vi "Vehicle Position Simulation View.vi"(8 "error in (no error)":errorcluster, 11 "View Model":T1) -> (0 "error out":errorcluster)   [LabVIEW 2017]
doc: "A software interface which mimics the hardware interfaces that communicate the vehicle position.\nUsed to simulate the travel of the car through the enclosure by activating Station sensors.\n[Covers: UI4]"
uses:
  View Model/Controls/View Model.ctl
  View Model/Controls/Shared Model.ctl
  Error Handler/Controls/Error Model.ctl
  Error Handler/Controls/Error Message.ctl
  Error Handler/Controls/Error Level.ctl
  Configuration/Controls/Database Model.ctl
  Configuration/Controls/Database Message.ctl
  Configuration/Controls/Database Command.ctl
  Configuration/Controls/Database Overhead.ctl
  Configuration/Controls/Database Status.ctl
  Configuration/Controls/Database Record.ctl
  Configuration/Controls/Database - Rule Record.ctl
  Controller/Controls/CNTRLR - Wash Step.ctl
  Controller/Controls/CNTRLR - Position.ctl
  Controller/Controls/CNTRLR - Model.ctl
  Controller/Controls/CNTRLR - Message.ctl
  Controller/Controls/CNTRLR - Command.ctl
  Controller/Controls/CNTRLR - Overhead.ctl
  Controller/Controls/CNTRLR - State.ctl
panel:
  in  "Position":u32(slide) caption="Vehicle Position Simulation" max=4 scale=0.0..4.0
  # "[Covers: UI4A]"
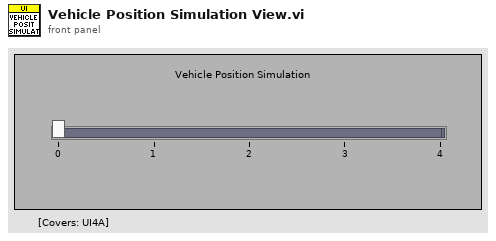
[diagram p1: front panel]
types:
  T1 = typedef "View Model.ctl" = cluster{"Shared Model":T2, "Error Model":T3, "DB Model":T4, "CNTRLR Model":T5}
  T2 = typedef "Shared Model.ctl" = cluster{"Stop":refnum<user-event>, "Stop DVR":refnum<data-value>}
  T3 = typedef "Error Model.ctl" = cluster{"Error Message":refnum<user-event>}
  T4 = typedef "Database Model.ctl" = cluster{"DB Message":refnum<user-event>, "DB Overhead DVR":refnum<data-value>}
  T5 = typedef "CNTRLR - Model.ctl" = cluster{"Message":refnum<user-event>, "Overhead DVR":refnum<data-value>, "Wash Entry":refnum<user-event>, "Out of Position":refnum<user-event>}
  T6 = typedef "CNTRLR - Position.ctl" = enum16{"Entry", "Station 1", "Station 2", "Station 3", "Exit"}
  T7 = typedef "CNTRLR - State.ctl" = enum16{"Initial", "Wait for Start", "Start State", "Wait for Vehicle Position", "Wash Step Execution", "Wash Step/Cycle Complete", "Wash Exit", "Wash Abort/Terminate"}
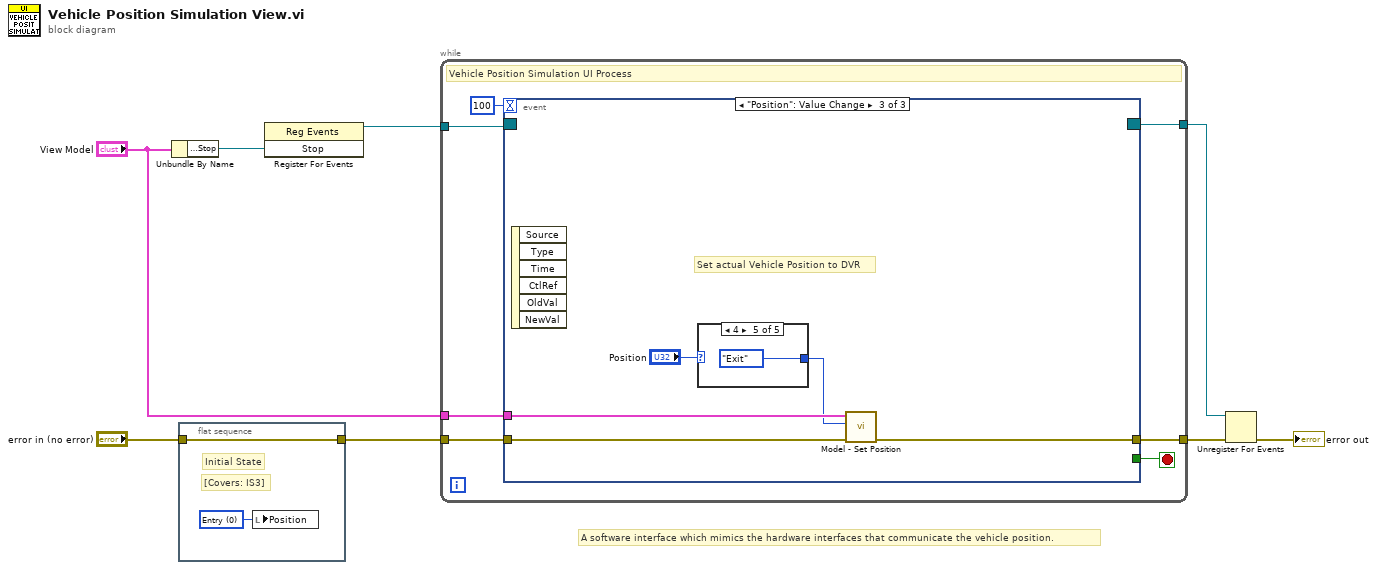
[diagram p0: block diagram]
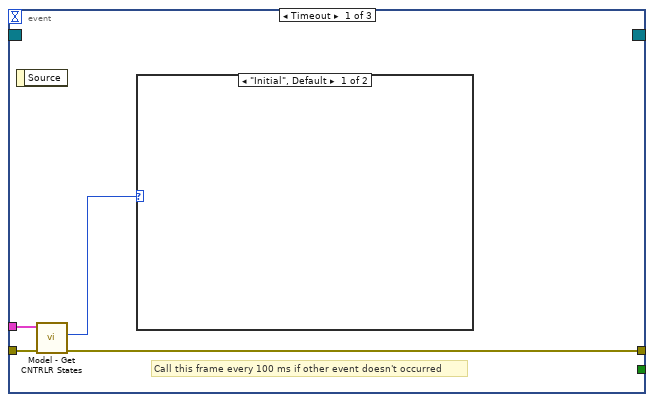
[diagram p2: hidden frame]
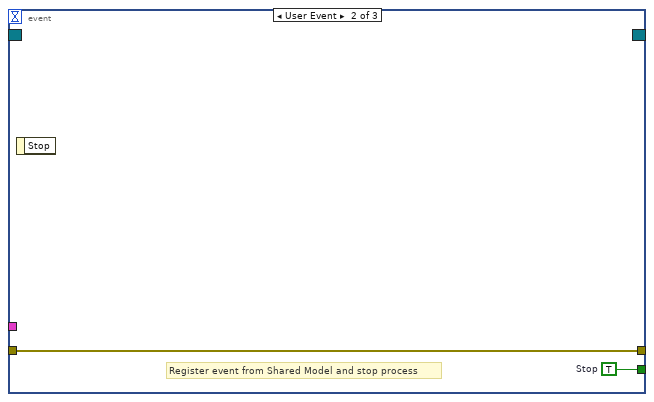
[diagram p4: hidden frame]
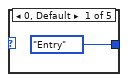
[diagram p5: hidden frame]
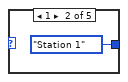
[diagram p6: hidden frame]
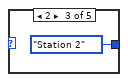
[diagram p7: hidden frame]
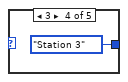
[diagram p8: hidden frame]
diagram:
  # "A software interface which mimics the hardware interfaces that communicate the vehicle position."
  n1 = Unbundle By Name("View Model") -> ("Shared Model.Stop"=w8:refnum<user-event>)
  n2 = flat-sequence {
    tunnel: "error in (no error)" -> [w10]
    tunnel: [w10] -> w1
    frame #0 {
      w9 = u32 0 items=["Entry", "Station 1", "Station 2", "Station 3", "Exit"] ("Position")
      # "[Covers: IS3]"
      # "Initial State"
      n3 = local write "Position"(w9) -> ()
    }
  }
  n4 = register-events(w8) -> (reference out=w7:refnum<event-registration>)  [unwired: 2 in, 1 out]
  n5 = while {
    tunnel: w7 -> [w17]
    tunnel: w1 -> [w16]
    tunnel: [w15] -> w5
    tunnel: [w12] -> w6
    tunnel: "View Model" -> [w11]
    stop <- w13 stop-if-true
    # "Vehicle Position Simulation UI Process"
    n6 = event shown="[2] \"Position\": Value Change" {
      selector: w17 -> [_ _ _]
      dyn-events: [_ _ _] -> w12
      timeout: 100 -> [_ _ _]
      tunnel: w16 -> [w21 w22 w27]
      tunnel: [w20 w22 w26] -> w15
      tunnel: [_ w23 _] -> w13
      tunnel: w11 -> [w19 _ w25]
      event Timeout {
        # "Call this frame every 100 ms if other event doesn't occurred"
        n7 = event-data() -> ()  [unwired: 1 in, 1 out]
        n8 = call "Model - Get CNTRLR States.vi"("error in (no error)"=w21, "View Model"=w19) -> ("error out"=w20:errorcluster, "Current State"=w18:T7)  [unwired: 6 in, 2 out]
        n9 = case shown="\"Initial\", Default" w18 {
          frame "Initial", Default {
          }
          frame "Wait for Start" {
          }
        }
      }
      event User Event {
        w23 = TRUE  # Stop
        # "Register event from Shared Model and stop process"
        n10 = event-data() -> ()  [unwired: 1 in, 1 out]
      }
      event "Position": Value Change {
        # "Set actual Vehicle Position to DVR"
        n11 = event-data() -> ()  [unwired: 1 in, 6 out]
        n12 = case shown="4" "Position" {
          tunnel: [CNTRLR_-_Position."Entry" ("Vehicle Position") CNTRLR_-_Position."Station 1" ("Vehicle Position") CNTRLR_-_Position."Station 2" ("Vehicle Position") CNTRLR_-_Position."Station 3" ("Vehicle Position") CNTRLR_-_Position."Exit" ("Vehicle Position")] -> w24
          frame 0, Default {
          }
          frame 1 {
          }
          frame 2 {
          }
          frame 3 {
          }
          frame 4 {
          }
        }
        n13 = call "Model - Set Position.vi"("error in (no error)"=w27, "Vehicle Position"=w24, "View Model"=w25) -> ("error out"=w26:errorcluster)  [unwired: 7 in, 1 out]
      }
    }
  }
  n14 = Unregister For Events(event registration refnum=w6, error in=w5) -> (error out=→"error out":errorcluster)
